vi "Read Process Information (SubVI).vi"(8 "error in (no error)":errorcluster, 10 "Address":string, 11 "VISA Refnum in":refnum<visa-resource-name>) -> (0 "error out":errorcluster, 1 "PI String Array":T1, 2 "Received PI String":string, 3 "VISA Refnum out":refnum<visa-resource-name>, 6 "Error Text":string)   [LabVIEW 2020]
doc: "Reads Instrument Process Information [PI] data: Mass Flow, Volumetric Flow, Totalizer#1, Totalizer#2 , Gas Temperature, Gas Pressure, Flow Alarm Status, Temperature Alarm Status, Pressure Alarm Status, Alarm Events Register and Diagnostic Events Register. Returns array of strings.\nMass Flow Rate (MEU)\nVolumetric Flow Rate (VEU)\nTotalizer#1 value (MEU)\nTotalizer#2 value (MEU)\nGas Temperature (TEU)\nGas Pressure (PEU)\nFlow Alarm Status [D,N,H,L]\nTemp. Alarm Status [D,N,H,L]\nPress. Alarm Status [D,N,H,L]\nCurrent status of the Alarm Events Register (Hex, bitwise notation)\nCurrent status of Diagnostic Events Register (Hex, bitwise notation)\nNOTE: See list of the Alarm and Diagnostic Events in the instrument operating manual."
uses:
  <vilib>/Instr/_visa.llb/VISA Flush IO Buffer Mask.ctl
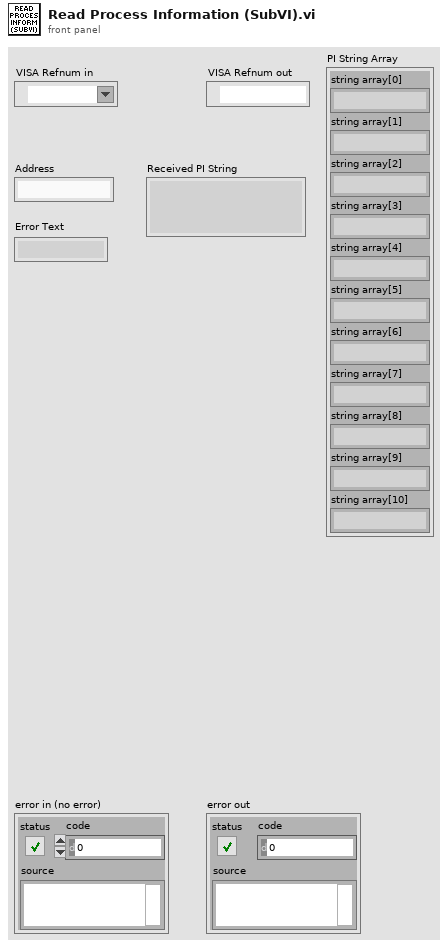
[diagram p1: front panel]
types:
  T1 = cluster{"string array[0]":string, "string array[1]":string, "string array[2]":string, "string array[3]":string, "string array[4]":string, "string array[5]":string, "string array[6]":string, "string array[7]":string, "string array[8]":string, "string array[9]":string, "string array[10]":string}
  T2 = typedef "VISA Flush IO Buffer Mask.ctl" = u16
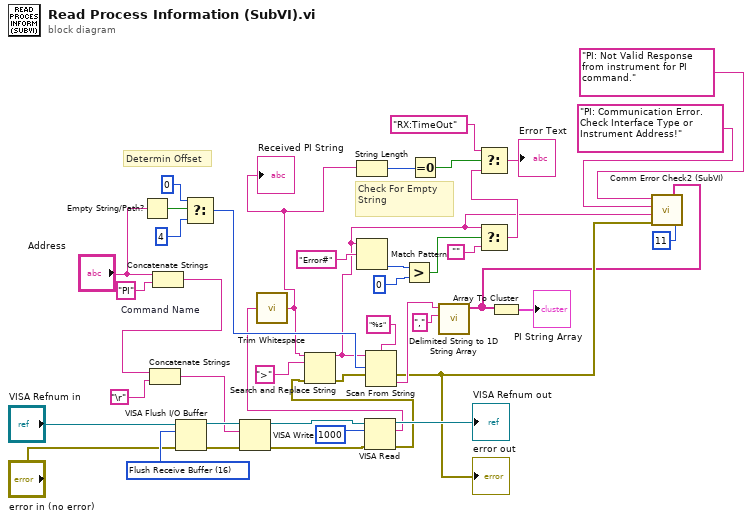
[diagram p0: block diagram]
diagram:
  w40 = "PI"  # Command Name
  w39 = T2 16 items=["Flush Receive Buffer"=16, "Write Transmit Buffer to Device"=32, "Flush Receive Buffer (No I/O)"=64, "Flush Transmit Buffer"=128] ("Mask")
  # "Check For Empty String"
  # "Determin Offset"
  n1 = Empty String/Path?(string/path="Address") -> (empty?=w23:bool)
  n2 = Concatenate Strings("Address", w40) -> (w41:string)
  n3 = Concatenate Strings(w41, "\r") -> (w32:string)
  n4 = VISA Flush I/O Buffer(VISA resource name="VISA Refnum in", mask (16)=w39, error in (no error)="error in (no error)") -> (VISA resource name out=w36:refnum<visa-resource-name>, error out=w37:errorcluster)
  n5 = Select(t=0, s=w23, f=4) -> (s? t:f=w16:i32)
  n6 = VISA Write(VISA resource name=w36, write buffer=w32, error in (no error)=w37) -> (VISA resource name out=w28:refnum<visa-resource-name>, error out=w30:errorcluster)  [unwired: 1 out]
  n7 = VISA Read(VISA resource name=w28, byte count=u32 1000, error in (no error)=w30) -> (VISA resource name out=→"VISA Refnum out":refnum<visa-resource-name>, read buffer=w9:string, error out=w18:errorcluster)  [unwired: 1 out]
  n8 = call <vilib>:"Trim Whitespace.vi"("string"=w9) -> ("trimmed string"=w7:string)  [unwired: 1 in]
  "Received PI String" <- w7
  n9 = Search and Replace String(input string=w7, search string=">", error in=w18) -> (result string=w2:string, error out=w17:errorcluster)  [unwired: 5 in, 2 out]
  n10 = String Length(string=w7) -> (length=w10:i32)
  n11 = Match Pattern(string=w2, regular expression="Error#") -> (offset past match=w25:i32)  [unwired: 1 in, 3 out]
  n12 = Scan From String(format string="%s", input string=w2, initial scan location=w16, error in=w17) -> (error out=w6:errorcluster, output 1=w15:string)  [unwired: 1 in, 2 out]
  "error out" <- w6
  n13 = Greater?(x=w25, y=0) -> (0:w24:bool)
  n14 = Equal To 0?(x=w10) -> (x = 0?=w14:bool)
  n15 = call <vilib>:"Delimited String to 1D String Array.vi"("delimiter"=",", "delimited string"=w15) -> ("string array"=w1:string[])  [unwired: 9 in]
  n16 = Select(t=w2, s=w24, f="") -> (s? t:f=w12:string)
  n17 = Select(t="RX:TimeOut", s=w14, f=w12) -> (s? t:f=→"Error Text":string)
  n18 = Array To Cluster(array=w1) -> (cluster=→"PI String Array":T1)
  n19 = call "Comm Error Check2 (SubVI).vi"("Number of Arguments"=11, "Reply string array"=w1, "error in (no error)"=w6, "Reply string"=w2, "Error Source String 2"="PI: Communication Error. Check Interface Type or Instrument Address!", "Error Source String 1"="PI: Not Valid Response from instrument for PI command.") -> ()
